vi "RXSTAT.vi"(0 "SPI Config In":T1) -> (1 "SPI Config Out":T1, 2 "Frames Read":u8[](array[numeric]))   [LabVIEW 2019]
uses:
  SPI/SPI Config.ctl
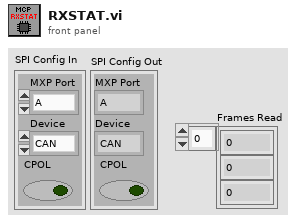
[diagram p1: front panel]
types:
  T1 = typedef "SPI Config.ctl" = cluster{"MXP Port":enum16{"A", "B"}, "Device":enum16{"CAN", "ENC", "IMU1", "IMU2"}, "CPOL":bool}
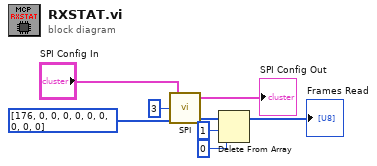
[diagram p0: block diagram]
diagram:
  n1 = call "SPI.vi"("Data to Write"=u8[] [176, 0, 0, 0, 0, 0, 0, 0, 0, 0], "Frames to Write"=u8 3, "SPI Config In"="SPI Config In") -> ("Data Read"=w4:u8[], "SPI Config Out"=→"SPI Config Out":T1)  [unwired: 1 out]
  n2 = Delete From Array(array=w4, length=1, index=0) -> (array with subset deleted=→"Frames Read":u8[])  [unwired: 1 out]
